vi "Toggle Node Selection.vi"(8 "error in (no error)":errorcluster, 9 "New selection":i32=-1, 11 "FSM in":refnum<class "FSM.Graph.lvclass">) -> (0 "error out":errorcluster, 3 "FSM out":refnum<class "FSM.Graph.lvclass">)   [LabVIEW 2015, in "FSM.Graph.lvclass"]
uses:
  FSM.Graph.lvclass
  FSM.Graph.lvclass/FSM.Graph.ctl
  FSM.Node/FSM.Node.lvclass/FSM.Node.ctl
  FSM.Node/Read selected.vi
  FSM.Node/Write selected.vi
  FSM.Node/FSM.Node.lvclass
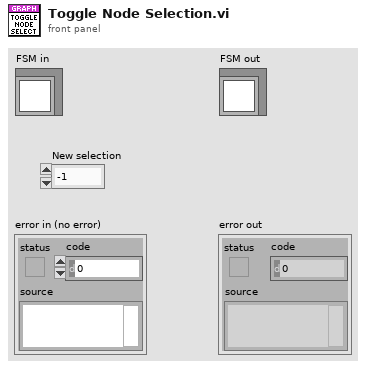
[diagram p1: front panel]
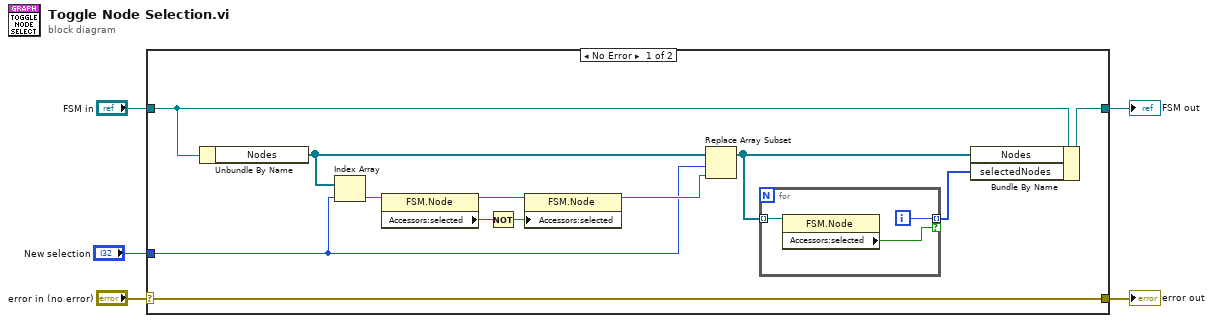
[diagram p0: block diagram]
diagram:
  n1 = case shown="No Error" "error in (no error)" {
    selector: "error in (no error)" -> [w17 w22]
    tunnel: [w17 w22] -> w4
    tunnel: [w15 w21] -> w2
    tunnel: "FSM in" -> [w16 w21]
    tunnel: "New selection" -> [w8 _]
    frame No Error {
      n2 = Unbundle By Name(w16) -> ("Nodes"=w10:refnum<class "FSM.Node.lvclass">[])
      n3 = Index Array(array=w10, index=w8) -> (element=w14:refnum<class "FSM.Node.lvclass">)
      n4 = property class="FSM.Node"(reference=w14) -> (reference out=w12:refnum<class "FSM.Node.lvclass">, "Accessors:selected"=w13:bool)  [unwired: 1 in, 1 out]
      n5 = Not(x=w13) -> (.not. x?=w11:bool)
      n6 = property class="FSM.Node"(reference=w12, "Accessors:selected"=w11) -> (reference out=w9:refnum<class "FSM.Node.lvclass">)  [unwired: 1 in, 1 out]
      n7 = Replace Array Subset(array=w10, new element=w9, index=w8) -> (w7:refnum<class "FSM.Node.lvclass">[])
      n8 = for {
        tunnel: w7 -> [w20] mode=indexing
        tunnel: [w19] -> w6 mode=indexing if=w18
        i -> [w19]
        n9 = property class="FSM.Node"(reference=w20) -> ("Accessors:selected"=w18:bool)  [unwired: 1 in, 2 out]
      }
      n10 = Bundle By Name(cluster=w16, "Nodes"=w7, "selectedNodes"=w6) -> (w15:refnum<class "FSM.Graph.lvclass">)
    }
    frame Error {
    }
  }
  "error out" <- w4
  "FSM out" <- w2
